vi "提取仪器参数 (子VI).vi"(10 "因子编码":string, 11 "数据输入":string[](array[string])) -> (3 "字符串":string)   [LabVIEW 2016, in "数据传输系统.lvlib"]
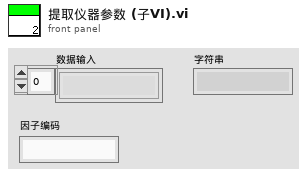
[diagram p1: front panel]
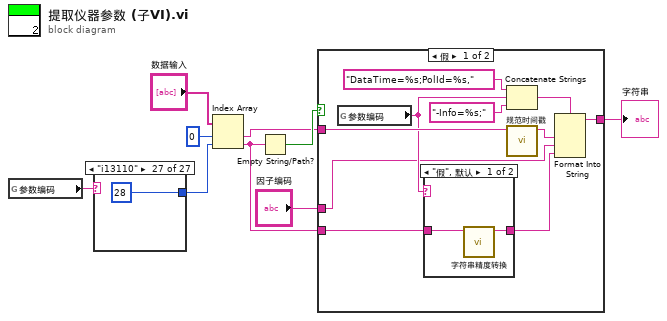
[diagram p0: block diagram]
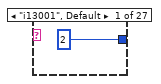
[diagram p2: hidden frame]
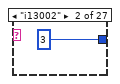
[diagram p3: hidden frame]
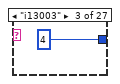
[diagram p4: hidden frame]
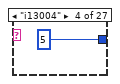
[diagram p5: hidden frame]
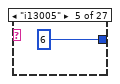
[diagram p6: hidden frame]
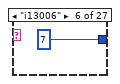
[diagram p7: hidden frame]
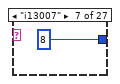
[diagram p8: hidden frame]
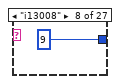
[diagram p9: hidden frame]
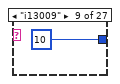
[diagram p10: hidden frame]
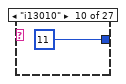
[diagram p11: hidden frame]
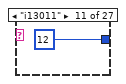
[diagram p12: hidden frame]
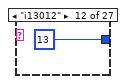
[diagram p13: hidden frame]
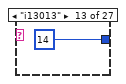
[diagram p14: hidden frame]
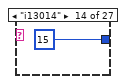
[diagram p15: hidden frame]
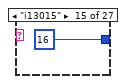
[diagram p16: hidden frame]
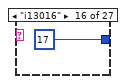
[diagram p17: hidden frame]
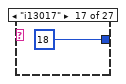
[diagram p18: hidden frame]
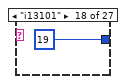
[diagram p19: hidden frame]
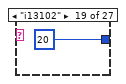
[diagram p20: hidden frame]
diagram:
  n1 = global read "全局 提取仪器参数.vi" "参数编码"() -> (w8:string)
  n2 = case shown="\"i13110\"" w8 {
    tunnel: [2 ("索引") 3 ("索引") 4 ("索引") 5 ("索引") 6 ("索引") 7 ("索引") 8 ("索引") 9 ("索引") 10 ("索引") 11 ("索引") 12 ("索引") 13 ("索引") 14 ("索引") 15 ("索引") 16 ("索引") 17 ("索引") 18 ("索引") 19 ("索引") 20 ("索引") 21 ("索引") 22 ("索引") 23 ("索引") 24 ("索引") 25 ("索引") 26 ("索引") 27 ("索引") 28 ("索引")] -> w9
    frame "i13001", Default {
    }
    frame "i13002" {
    }
    frame "i13003" {
    }
    frame "i13004" {
    }
    frame "i13005" {
    }
    frame "i13006" {
    }
    frame "i13007" {
    }
    frame "i13008" {
    }
    frame "i13009" {
    }
    frame "i13010" {
    }
    frame "i13011" {
    }
    frame "i13012" {
    }
    frame "i13013" {
    }
    frame "i13014" {
    }
    frame "i13015" {
    }
    frame "i13016" {
    }
    frame "i13017" {
    }
    frame "i13101" {
    }
    frame "i13102" {
    }
    frame "i13103" {
    }
    frame "i13104" {
    }
    frame "i13105" {
    }
    frame "i13106" {
    }
    frame "i13107" {
    }
    frame "i13108" {
    }
    frame "i13109" {
    }
    frame "i13110" {
    }
  }
  n3 = Index Array(array="数据输入", index #1=0 ("索引"), index #2=w9) -> (element #1=w3:string, element #2=w2:string)
  n4 = Empty String/Path?(string/path=w2) -> (empty?=w4:bool)
  n5 = case shown="假" w4 {
    tunnel: [w45 ""] -> w7
    tunnel: w3 -> [w44 _]
    tunnel: w2 -> [w39 _]
    tunnel: "因子编码" -> [w37 _]
    frame False {
      n6 = global read "全局 提取仪器参数.vi" "参数编码"() -> (w40:string)
      n7 = case shown="\"假\", 默认" w40 {
        tunnel: w39 -> [w48 w50]
        tunnel: [w47 w49] -> w38
        frame "假", Default {
          n8 = call "字符串精度转换.vi"("输入字符串"=w48) -> ("输出字符串"=w47:string)  [unwired: 9 in, 1 out]
        }
        frame "i13006", "i13013" {
          n9 = call "规范时间戳.vi"("字符串"=w50) -> ("result string"=w49:string)  [unwired: 10 in]
        }
      }
      n10 = Concatenate Strings("DataTime=%s;PolId=%s," ("格式字符串"), w40, "-Info=%s;" ("格式字符串")) -> (w41:string)
      n11 = call "规范时间戳.vi"("字符串"=w44) -> ("result string"=w46:string)  [unwired: 10 in]
      n12 = Format Into String(format string=w41, w46, w37, w38) -> (resulting string=w45:string)  [unwired: 2 in, 1 out]
    }
    frame True {
    }
  }
  "字符串" <- w7
